vi "main.vi"() -> ()   [LabVIEW 2020]
uses:
  Traffic Signal.ctl
  Grade Gate.ctl
  PedX Signal.ctl
  Global Indicators.vi
panel:
  out "PedX 8":T1
  out "PedX 7":T1
  out "PedX 6":T1
  out "PedX 5":T1
  out "PedX 4":T1
  out "PedX 3":T1
  out "PedX 2":T1
  out "PedX":T1
  out "Grade Gate East":T2
  out "Grade Gate West":T2
  out "Nothbound":T3
  out "Westbound":T3
  out "Southbound":T3
  out "Eastbound":T3
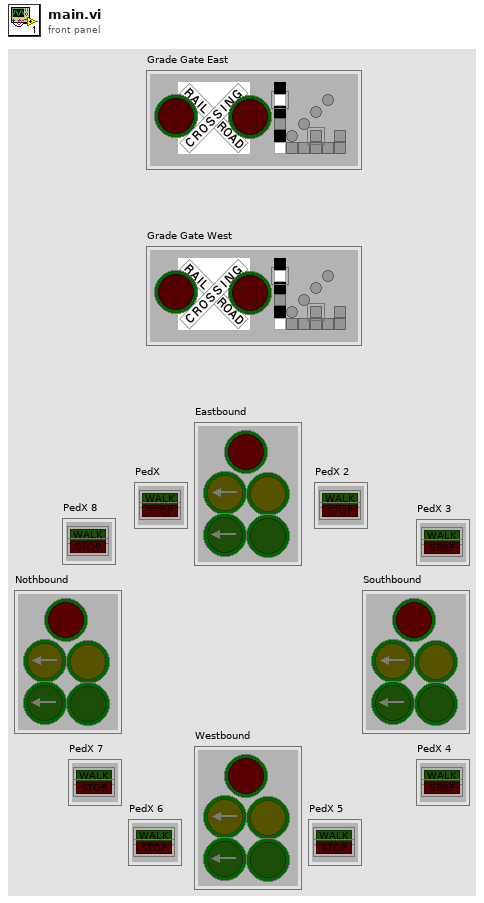
[diagram p1: front panel]
types:
  T1 = typedef "PedX Signal.ctl" = cluster{"PedX Walk":bool, "PedX Stop":bool}
  T2 = typedef "Grade Gate.ctl" = cluster{"UP 2":bool, "Pivot":bool, "UP 3":bool, "UP 4":bool, "UP 5":bool, "UP 6":bool, "DOWN 2":bool, "DOWN 3":bool, "DOWN 4":bool, "DOWN 5":bool, "DOWN 6":bool, "DOWN 7":bool, "DOWN 8":bool, "SIDE 2":bool, "SIDE 3":bool, "SIDE 4":bool, "SIDE 5":bool, "Blinky 2":bool, "Blinky 1":bool}
  T3 = typedef "Traffic Signal.ctl" = cluster{"Red Light":bool, "Yellow Light":bool, "Green Light":bool, "Yellow Turn":bool, "Green Turn":bool}
  T4 = enum16{"Resting", "Cycle", "Cycle PedX", "Train Approach", "911 Vehicle"}
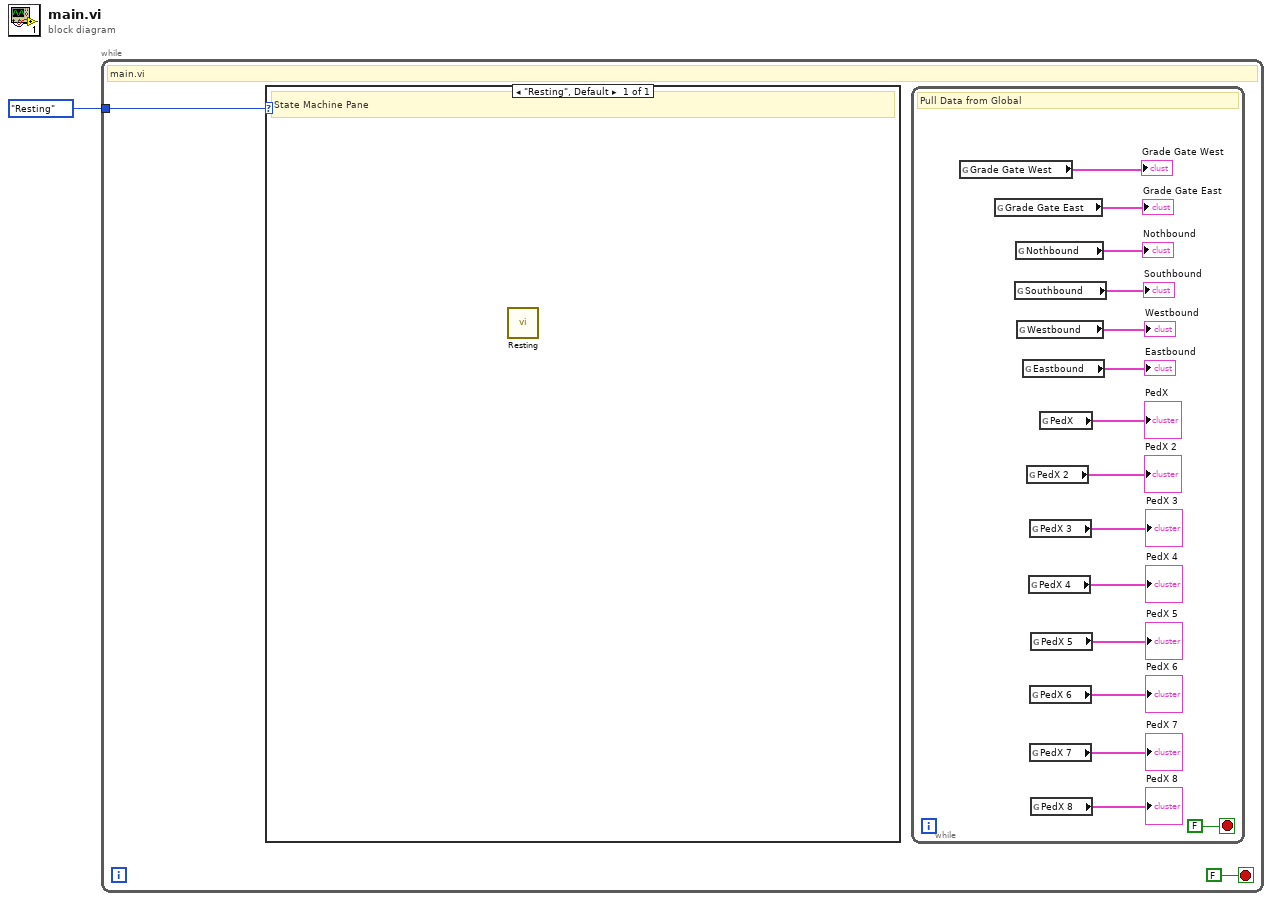
[diagram p0: block diagram]
diagram:
  n1 = while {
    tunnel: T4."Resting" -> [w3]
    stop <- FALSE stop-if-true
    # "main.vi"
    n2 = case shown="\"Resting\", Default" w3 {
      frame "Resting", Default {
        # "State Machine Pane"
        n3 = call "Resting.vi"() -> ()  [unwired: 1 in, 8 out]
      }
    }
    n4 = while {
      stop <- FALSE stop-if-true
      # "Pull Data from Global"
      n5 = global read "Global Indicators.vi" "Grade Gate West"() -> (→"Grade Gate West":T2)
      n6 = global read "Global Indicators.vi" "Grade Gate East"() -> (→"Grade Gate East":T2)
      n7 = global read "Global Indicators.vi" "Southbound"() -> (→"Southbound":T3)
      n8 = global read "Global Indicators.vi" "Nothbound"() -> (→"Nothbound":T3)
      n9 = global read "Global Indicators.vi" "Westbound"() -> (→"Westbound":T3)
      n10 = global read "Global Indicators.vi" "Eastbound"() -> (→"Eastbound":T3)
      n11 = global read "Global Indicators.vi" "PedX 2"() -> (→"PedX 2":T1)
      n12 = global read "Global Indicators.vi" "PedX 4"() -> (→"PedX 4":T1)
      n13 = global read "Global Indicators.vi" "PedX 3"() -> (→"PedX 3":T1)
      n14 = global read "Global Indicators.vi" "PedX 6"() -> (→"PedX 6":T1)
      n15 = global read "Global Indicators.vi" "PedX 7"() -> (→"PedX 7":T1)
      n16 = global read "Global Indicators.vi" "PedX 5"() -> (→"PedX 5":T1)
      n17 = global read "Global Indicators.vi" "PedX 8"() -> (→"PedX 8":T1)
      n18 = global read "Global Indicators.vi" "PedX"() -> (→"PedX":T1)
    }
  }
